vi "Input Cycle.vi"(8 "error in (no error)":errorcluster, 11 "RDS Local Remote Actor in":refnum<class "RDS Local Remote Actor.lvclass">) -> (0 "error out":errorcluster, 3 "RDS Local Remote Actor out":refnum<class "RDS Local Remote Actor.lvclass">)   [LabVIEW 2015, in "RDS Local Remote Actor.lvlib" / "RDS Local Remote Actor.lvclass"]
uses:
  RDS Local Remote Actor.lvclass
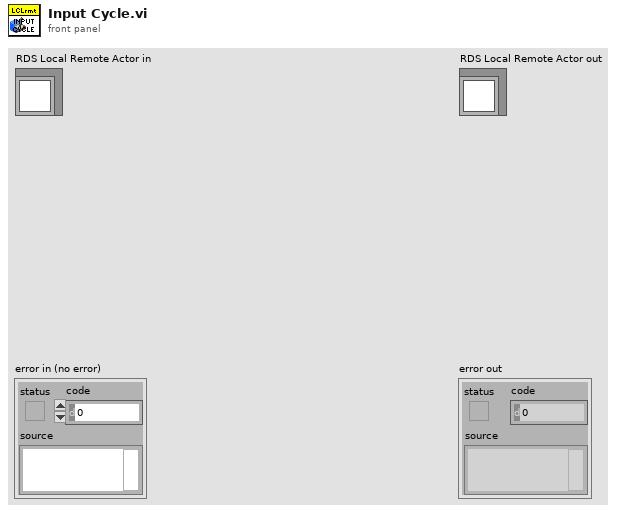
[diagram p1: front panel]
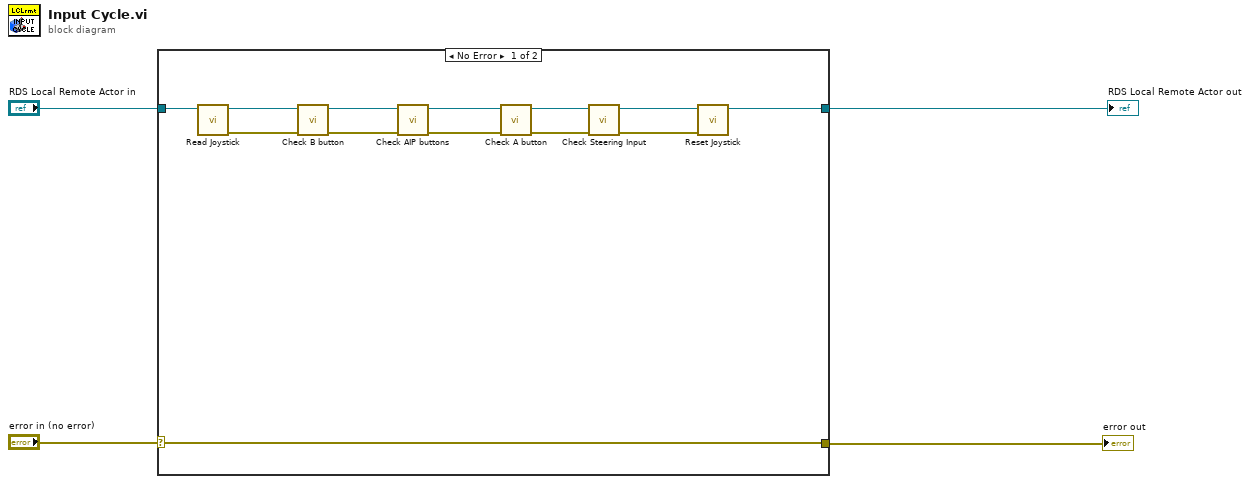
[diagram p0: block diagram]
diagram:
  n1 = case shown="No Error" "error in (no error)" {
    selector: "error in (no error)" -> [w17 w19]
    tunnel: [w17 w19] -> w3
    tunnel: [w11 w18] -> w1
    tunnel: "RDS Local Remote Actor in" -> [w16 w18]
    frame No Error {
      n2 = call "Read Joystick.vi"("RDS Local Remote Actor in"=w16) -> ("error out"=w15:errorcluster, "RDS Local Remote Actor out"=w14:refnum<class "RDS Local Remote Actor.lvclass">)  [unwired: 9 in]
      n3 = call "Check B button.vi"("error in (no error)"=w15, "RDS Local Remote Actor in"=w14) -> ("error out"=w12:errorcluster, "RDS Local Remote Actor out"=w13:refnum<class "RDS Local Remote Actor.lvclass">)  [unwired: 8 in]
      n4 = call "Check AIP buttons.vi"("error in (no error)"=w12, "RDS Local Remote Actor in"=w13) -> ("error out"=w7:errorcluster, "RDS Local Remote Actor out"=w10:refnum<class "RDS Local Remote Actor.lvclass">)  [unwired: 8 in]
      n5 = call "Check A button.vi"("error in (no error)"=w7, "RDS Local Remote Actor in"=w10) -> ("error out"=w6:errorcluster, "RDS Local Remote Actor out"=w9:refnum<class "RDS Local Remote Actor.lvclass">)  [unwired: 8 in]
      n6 = call "Check Steering Input.vi"("error in (no error)"=w6, "RDS Local Remote Actor in"=w9) -> ("error out"=w5:errorcluster, "RDS Local Remote Actor out"=w8:refnum<class "RDS Local Remote Actor.lvclass">)  [unwired: 8 in]
      n7 = call "Reset Joystick.vi"("error in (no error)"=w5, "RDS Local Remote Actor in"=w8) -> ("RDS Local Remote Actor out"=w11:refnum<class "RDS Local Remote Actor.lvclass">)  [unwired: 8 in, 1 out]
    }
    frame Error {
    }
  }
  "error out" <- w3
  "RDS Local Remote Actor out" <- w1
